vi "Convert Relative Path.vi"(10 "File Path in":path) -> (2 "Modified Path":path)   [LabVIEW 2020, in "Reports.lvlib" / "Report.lvclass"]
doc: "If a relative path, convert to the full directory.\n\n<b>Developed by:</b>\nDaniel Coons, TSC"
uses:
  Report.lvclass
  Report.lvclass/Report.ctl
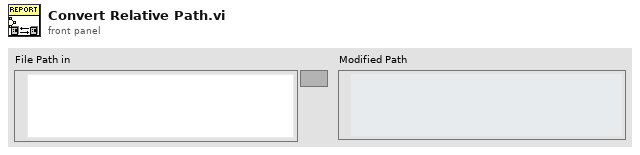
[diagram p1: front panel]
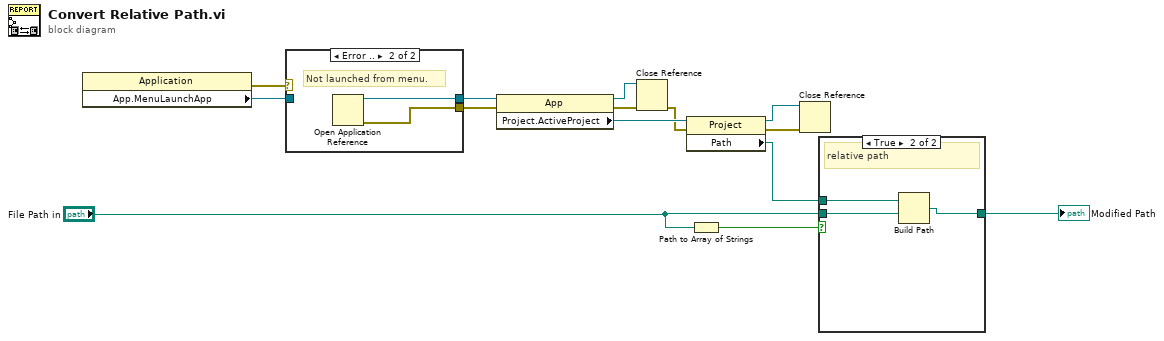
[diagram p0: block diagram]
diagram:
  n1 = property class="Application"() -> (error out=w1:errorcluster, "App.MenuLaunchApp"=w2:refnum<vi>)  [unwired: 2 in, 1 out]
  n2 = case shown="Error .." w1 {
    selector: w1 -> [w15 _]
    tunnel: [w16 w18] -> w4
    tunnel: w2 -> [w16 _]
    tunnel: [w15 w17] -> w7
    frame No Error {
      # "Launch from menu"
    }
    frame Error {
      # "Not launched from menu."
      n3 = Open Application Reference() -> (0:w17:errorcluster, 3:w18:refnum<vi>)  [unwired: 4 in]
    }
  }
  n4 = property class="App"(reference=w4, error in=w7) -> (reference out=w6:refnum<vi>, error out=w8:errorcluster, "Project.ActiveProject"=w5:refnum<vi>)
  n5 = Close Reference(reference=w6, error in (no error)=w8) -> (error out=w3:errorcluster)
  n6 = property class="Project"(reference=w5, error in=w3) -> (reference out=w9:refnum<vi>, error out=w10:errorcluster, "Path"=w11:path)
  n7 = Path to Array of Strings(0:"File Path in") -> (1:w14:bool)  [unwired: 1 out]
  n8 = Close Reference(reference=w9, error in (no error)=w10) -> ()  [unwired: 1 out]
  n9 = case shown="True" w14 {
    tunnel: "File Path in" -> [w19 w20]
    tunnel: [w19 w21] -> w12
    tunnel: w11 -> [_ w22]
    frame False {
      # "absolute path"
    }
    frame True {
      # "relative path"
      n10 = Build Path(base path=w22, name or relative path=w20) -> (appended path=w21:path)
    }
  }
  "Modified Path" <- w12
